vi "Update Dashboard.vi"   [LabVIEW 2013]
uses:
  Team Code/Robot Global Data.vi
types:
  T1 = cluster{"Motor Divide":dbl, "Use Gamepad Drive":bool, "Use Linearity Drive":bool, "Use Gamepad Arm":bool, "Average FPS":dbl, "Gamepad Tank Drive?":bool, "Run Autonomous?":bool, "Average Distance":dbl, "Remus?":bool}
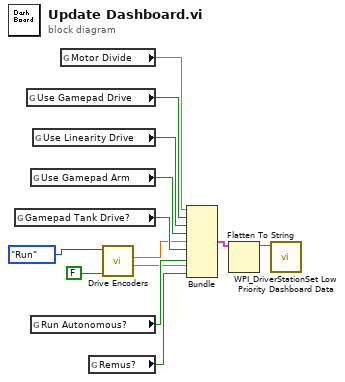
[diagram p0: block diagram]
diagram:
  n1 = global read "Robot Global Data.vi" "Gamepad Tank Drive?"() -> (w7:bool)
  n2 = global read "Robot Global Data.vi" "Use Gamepad Drive"() -> (w10:bool)
  n3 = global read "Robot Global Data.vi" "Use Gamepad Arm"() -> (w8:bool)
  n4 = global read "Robot Global Data.vi" "Run Autonomous?"() -> (w6:bool)
  n5 = global read "Robot Global Data.vi" "Use Linearity Drive"() -> (w9:bool)
  n6 = global read "Robot Global Data.vi" "Motor Divide"() -> (w11:dbl)
  n7 = global read "Robot Global Data.vi" "Remus?"() -> (w1:bool)
  n8 = call "Drive Encoders.vi"("Reset Encoders?"=FALSE, "Mode"=enum16{"Init", "Run", "End"}."Run") -> ("Average Distance"=w3:dbl, "Average FPS"=w2:dbl)  [unwired: 2 in, 6 out]
  n9 = Bundle("Motor Divide"=w11, "Use Gamepad Drive"=w10, "Use Linearity Drive"=w9, "Use Gamepad Arm"=w8, "Average FPS"=w2, "Gamepad Tank Drive?"=w7, "Run Autonomous?"=w6, "Average Distance"=w3, "Remus?"=w1) -> (w12:T1)  [unwired: 1 out]
  n10 = Flatten To String(anything=w12) -> (data string=w13:string)  [unwired: 1 in, 4 out]
  n11 = call <vilib>:"WPI_DriverStationSet Low Priority Dashboard Data.vi"("User Data"=w13) -> ()  [unwired: 1 in, 10 out]
